vi "Organize Aliases by Module.vi"(11 "Alias Mappings":T2[](array[typedef])) -> (3 "Mappings by Module":T1(array[cluster]))   [LabVIEW 2017, in "Routing and Faulting System Explorer.lvlib"]
uses:
  Routing and Faulting System Explorer.lvlib
  Shared/Alias Mapping.ctl
  Shared/Routing and Faulting Shared.lvlib
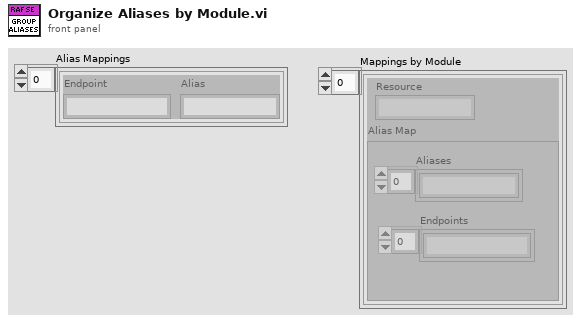
[diagram p1: front panel]
types:
  T1 = cluster{"Resource":string, "Alias Map":cluster{"Aliases":string[], "Endpoints":string[]}}[]
  T2 = typedef "Routing and Faulting Shared.lvlib/Alias Mapping.ctl" = cluster{"Endpoint":string, "Alias":string}
  T3 = cluster{"Resource":string, "Alias Map":cluster{"Aliases":string[], "Endpoints":string[]}}
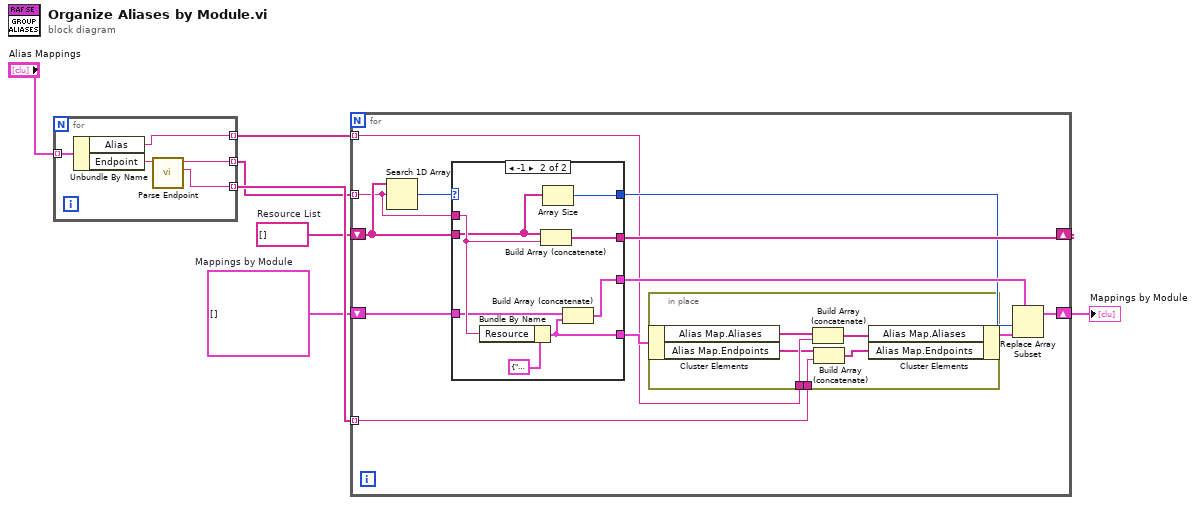
[diagram p0: block diagram]
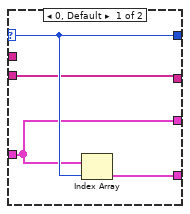
[diagram p2: hidden frame]
diagram:
  w2 = T1 []  # Mappings by Module
  w3 = string[] []  # Resource List
  n1 = for {
    tunnel: "Alias Mappings" -> [w12] mode=indexing
    tunnel: [w10] -> w4 mode=indexing
    tunnel: [w9] -> w5 mode=indexing
    tunnel: [w8] -> w6 mode=indexing
    n2 = Unbundle By Name(w12) -> ("Alias"=w8:string, "Endpoint"=w11:string)
    n3 = call "Parse Endpoint.vi"("Resource/Endpoint"=w11) -> ("Endpoint"=w9:string, "Resource"=w10:string)  [unwired: 9 in]
  }
  n4 = for {
    shift-right: [w20] -> _
    shift-left: w3 -> [w23]
    tunnel: w4 -> [w21] mode=indexing
    shift-right: [w15] -> w1
    shift-left: w2 -> [w22]
    tunnel: w5 -> [w13] mode=indexing
    tunnel: w6 -> [w14] mode=indexing
    n5 = Search 1D Array(1D array=w23, element=w21) -> (index of element=w24:i32)  [unwired: 1 in]
    n6 = case shown="-1" w24 {
      selector: w24 -> [w34 _]
      tunnel: w23 -> [w32 w40]
      tunnel: w22 -> [w31 w38]
      tunnel: w21 -> [_ w42]
      tunnel: [w33 w37] -> w19
      tunnel: [w32 w41] -> w20
      tunnel: [w34 w39] -> w17
      tunnel: [w31 w36] -> w18
      frame 0, Default {
        n7 = Index Array(array=w31, index=w34) -> (element=w33:T3)
      }
      frame -1 {
        n8 = Bundle By Name(cluster=T3 {"Resource"="", "Alias Map"={"Aliases"=[], "Endpoints"=[]}} ("Alias Mappings"), "Resource"=w42) -> (w37:T3)
        n9 = Build Array (concatenate)(w40, w42) -> (w41:string[])
        n10 = Array Size(array=w40) -> (size(s)=w39:i32)
        n11 = Build Array (concatenate)(w38, w37) -> (w36:T1)
      }
    }
    n12 = in-place {
      in-place-border: w14 -> [w28]
      in-place-border: w13 -> [w26]
      n13 = in-place-cluster #1(w19) -> ("Alias Map.Aliases"=w30:string[], "Alias Map.Endpoints"=w27:string[])
      n14 = Build Array (concatenate)(w30, w28) -> (w29:string[])
      n15 = Build Array (concatenate)(w27, w26) -> (w25:string[])
      n16 = in-place-cluster #1("Alias Map.Aliases"=w29, "Alias Map.Endpoints"=w25) -> (w16:T3)
    }
    n17 = Replace Array Subset(array=w18, new element=w16, index=w17) -> (w15:T1)
  }
  "Mappings by Module" <- w1
